vi "Read Key (Boolean).vi"(7 "Section Name":string, 8 "error in (no error)":errorcluster, 9 "Default":bool, 10 "Key Name":string, 11 "Config in":refnum<class "LabVIEW-Config.lvclass">) -> (0 "error out":errorcluster, 1 "Value":bool, 2 "Key Found?":bool, 3 "Config out":refnum<class "LabVIEW-Config.lvclass">)   [LabVIEW 2017, in "LabVIEW-Config.lvlib" / "LabVIEW-Config.lvclass"]
uses:
  LabVIEW-Config.lvclass
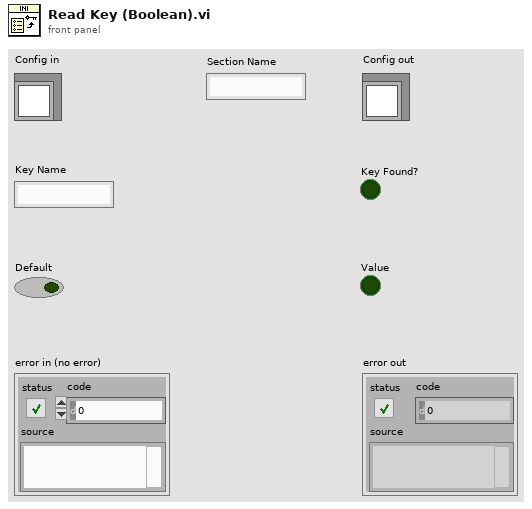
[diagram p1: front panel]
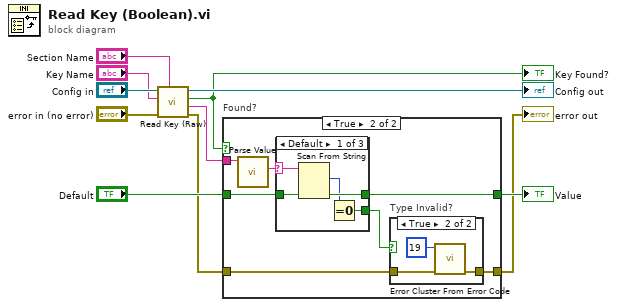
[diagram p0: block diagram]
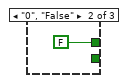
[diagram p3: hidden frame]
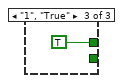
[diagram p4: hidden frame]
diagram:
  n1 = call "Read Key (Raw).vi"("Section Name"="Section Name", "error in (no error)"="error in (no error)", "Key Name"="Key Name", "Config in"="Config in") -> ("error out"=w2:errorcluster, "Content"=w6:string, "Key Found?"=w1:bool, "Config out"=→"Config out":refnum<class "LabVIEW-Config.lvclass">)  [unwired: 4 in]
  "Key Found?" <- w1
  n2 = case "Found?" shown="True" w1 {
    tunnel: w6 -> [_ w20]
    tunnel: [w13 w18] -> w5
    tunnel: "Default" -> [w13 w17]
    tunnel: [w12 w16] -> w3
    tunnel: w2 -> [w12 w14]
    frame False {
    }
    frame True {
      n3 = call "Parse Value.vi"("Value"=w20) -> ("Value (Comment Removed)"=w19:string)  [unwired: 9 in, 1 out]
      n4 = case shown="Default" w19 {
        selector: w19 -> [w25 _ _]
        tunnel: [w24 FALSE TRUE] -> w18
        tunnel: [w22 _ _] -> w15
        tunnel: w17 -> [w21 _ _]
        frame Default {
          n5 = Scan From String(input string=w25, default 1=w21) -> (offset past scan=w23:u32, output 1=w24:bool)  [unwired: 3 in, 2 out]
          n6 = Equal To 0?(x=w23) -> (x = 0?=w22:bool)
        }
        frame "0", "False" {
        }
        frame "1", "True" {
        }
      }
      n7 = case "Type Invalid?" shown="True" w15 {
        tunnel: w14 -> [w28 w30]
        tunnel: [w28 w29] -> w16
        frame False {
        }
        frame True {
          n8 = call <vilib>:"Error Cluster From Error Code.vi"("error in (no error)"=w30, "error code (0)"=19 ("Type invalid")) -> ("error out"=w29:errorcluster)  [unwired: 7 in]
        }
      }
    }
  }
  "error out" <- w3
  "Value" <- w5
